vi "Node Config.vi"(11 "VolatusAPI in":refnum<class "VolatusAPI.lvclass">) -> (2 "Node Config":refnum<class "Node Config.lvclass">, 3 "VolatusAPI out":refnum<class "VolatusAPI.lvclass">)   [LabVIEW 2020, in "Volatus.lvlib" / "VolatusAPI.lvclass"]
uses:
  VolatusAPI.lvclass
  VolatusConfig/Node/Node Config.lvclass
  VolatusAPI.lvclass/VolatusAPI.ctl
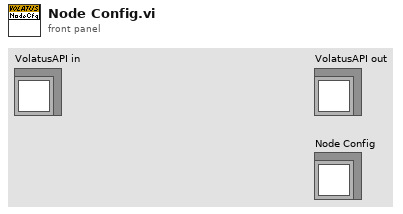
[diagram p1: front panel]
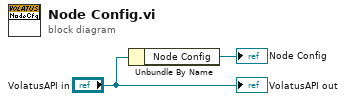
[diagram p0: block diagram]
diagram:
  n1 = Unbundle By Name("VolatusAPI in") -> ("Node Config"=→"Node Config":refnum<class "Node Config.lvclass">)
  "VolatusAPI out" <- "VolatusAPI in"
